vi "drivePID.vi"() -> ()   [LabVIEW 2013]
uses:
  State_Machine_Enum.ctl
  PCQueueDashboard/DBNameEnum.ctl
  RefnameEnum.ctl
  Robot Global Data.vi
  <vilib>/Rock Robotics/WPI/RobotDrive/WPI_RobotDriveGetSetRefNum.vi
panel:
  out "Loop Difference":u32
  in  "RPMRight":dbl(slide)=50.0 min=0.0 max=75.0 step=1.0 scale=0.0..75.0
  in  "RPMLeft":dbl(slide)=50.0 min=0.0 max=75.0 step=1.0 scale=0.0..75.0
  in  "output range RIGHT":cluster{"output high":dbl, "output low":dbl}={"output high"=1.0, "output low"=-1.0} {"output low" min=-1.0 max=1.0 step=0.1 format="%.2f"; "output high" min=-1.0 max=1.0 step=0.1 format="%.2f"}
  in  "output range LEFT":cluster{"output high":dbl, "output low":dbl}={"output high"=1.0, "output low"=-1.0} {"output low" min=-1.0 max=1.0 step=0.1 format="%.2f"; "output high" min=-1.0 max=1.0 step=0.1 format="%.2f"}
  in  "PID RIGHT":T1={"proportional gain (Kc)"=0.015, "integral time (Ti, min)"=0.001, "derivative time (Td, min)"=0.0} {"derivative time (Td, min)" format="%.3f"; "integral time (Ti, min)" format="%.3f"; "proportional gain (Kc)" format="%.3f"}
  in  "PID LEFT":T1={"proportional gain (Kc)"=0.015, "integral time (Ti, min)"=0.001, "derivative time (Td, min)"=0.0} {"derivative time (Td, min)" format="%.3f"; "integral time (Ti, min)" format="%.3f"; "proportional gain (Kc)" format="%.3f"}
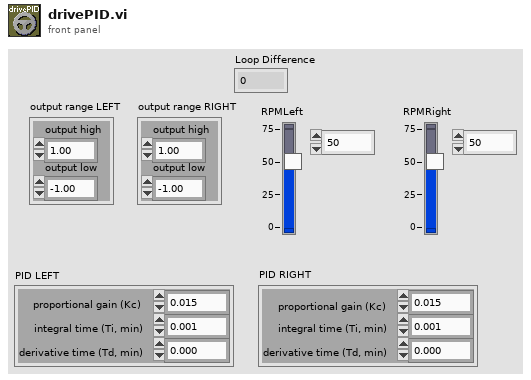
[diagram p1: front panel]
types:
  T1 = cluster{"proportional gain (Kc)":dbl, "integral time (Ti, min)":dbl, "derivative time (Td, min)":dbl}
  T2 = typedef "State_Machine_Enum.ctl" = enum16{"Idle", "Start", "Do", "Stop", "Init"}
  T3 = typedef "DBNameEnum.ctl" = enum16{"AutoInstructions", "DriveLoopTime", "DriveAlignLSLeft", "DriveAlignLSRight", "Use2DriveAlign", "ClimbLS", "LauncherAngleMatches", "FrameworkVersion", "sLauncherAngle", "LauncherTargetAngle", "sLauncherRPM", "LauncherTargetRPM", "sDriveDistance", "LauncherMotorValue", "PullbackTol", "FireTol", "LauncherRPMTol", "LauncherAngleTol", "InitialWait", "WaitBetweenLaunch", "AnglePresets", "RPMPresets", "UseAngleEncoder", "UseLauncherEncoder", "UseLauncherPID", "QSWaitBeforeFire", "QSWaitBeforeRetract", "AngleForwardValue", "AngleBackwardValue", "UseClusterArray", "BackupAuto", "ReverseDriveIndicate", "HalfSpeedFactor"}
  T4 = typedef "RefnameEnum.ctl" = enum16{"FireLauncher", "Climber", "Shield", "TankDrive", "DriveEncoderL", "DriveEncoderR", "LauncherMotorRPM", "LauncherEncoderAnalog", "LauncherEncoderRPM", "ShooterLS", "DriveAlignLSLeft", "DriveAlignLSRight", "ClimbingLS", "LauncherEncoderAngle", "LauncherMotorAngle", "Gamepad1", "Gamepad2", "Compressor", "ClimbWeightSol3", "ClimbWeightSol4"}
  T5 = typedef "WPI_DigitalInputDevRef.ctl" = cluster{"DevStatus":errorcluster, "DIO Channel":T6, "Digital Module":T7}
  T6 = typedef "FPGA_DIOChannel.ctl" = enum8{"DIO 1", "DIO 2", "DIO 3", "DIO 4", "DIO 5", "DIO 6", "DIO 7", "DIO 8", "DIO 9", "DIO 10", "DIO 11", "DIO 12", "DIO 13", "DIO 14", "Invalid"}
  T7 = typedef "FPGA_TypedefDigitalModule.ctl" = enum16{"Digital Module 1", "Digital Module 2"}
  T8 = typedef "WPI_RobotDriveDevRef.ctl" = cluster{"DevStatus":errorcluster, "Motors[]":T9[], "Square Inputs":bool, "Max Output":dbl, "Isochronous":bool}
  T9 = typedef "WPI_MotorControlDeviceRef.ctl" = cluster{"DeviceStatus":errorcluster, "Type":enum16{"PWM", "CAN"}, "PWM":cluster{"Digital Module":T7, "PWM Channel":T10, "DeadBand":T11}, "CAN":cluster{"Device Number":u8, "Control Mode":T12, "Semaphore":T13, "Max Vout":dbl}, "Invert":bool, "TransformRef":T14, "InvTransformRef":T14}
  T10 = typedef "FPGA_DIOPWMChannel.ctl" = enum8{"PWM 1", "PWM 2", "PWM 3", "PWM 4", "PWM 5", "PWM 6", "PWM 7", "PWM 8", "PWM 9", "PWM 10", "Invalid"}
  T11 = typedef "WPI_PWMDeadband.ctl" = cluster{"Name":string, "maxPositivePwm":i32, "minPositivePwm":i32, "centerPwm":i32, "maxNegativePwm":i32, "minNegativePwm":i32, "angularRange":u16}
  T12 = typedef "WPI_CANJaguar_ControlMode.ctl" = enum8{"Percent VBus", "Current", "Speed", "Position", "Voltage"}
  T13 = typedef "Semaphore RefNum" = refnum<k1>
  T14 = typedef "WPI_PWMTransform_ConPane.ctl" = refnum<vi>
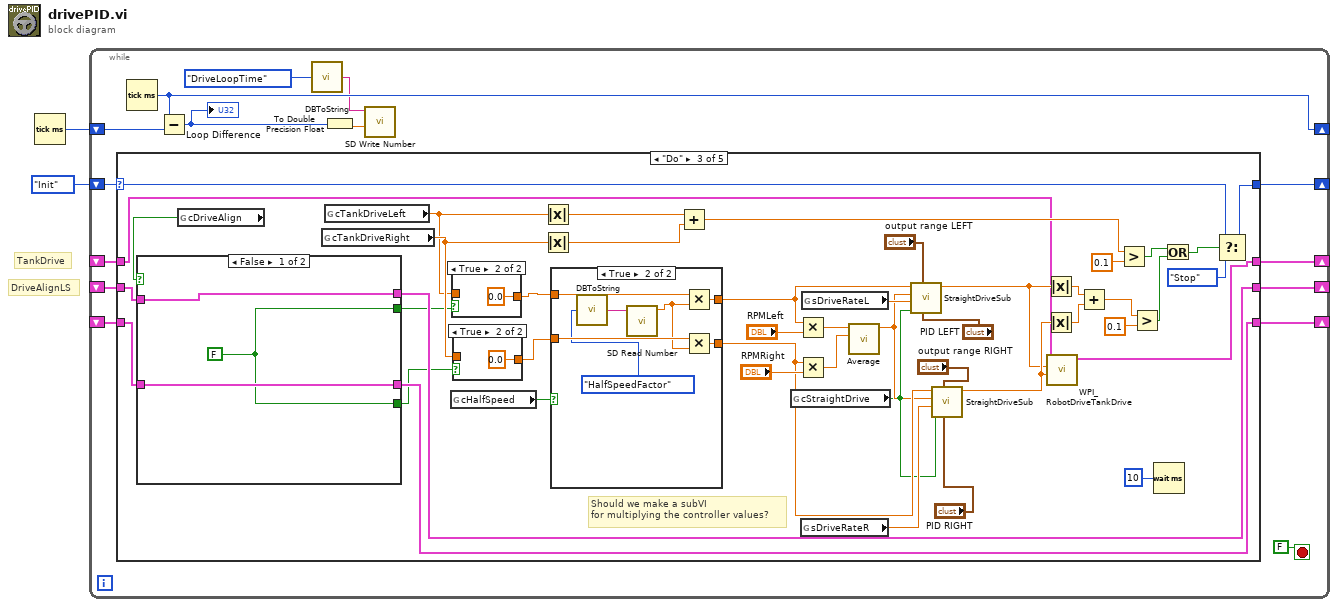
[diagram p0: block diagram]
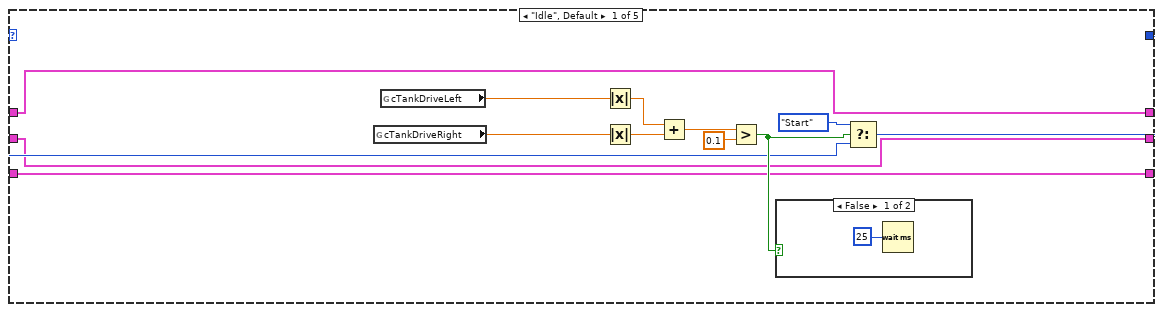
[diagram p2: hidden frame]
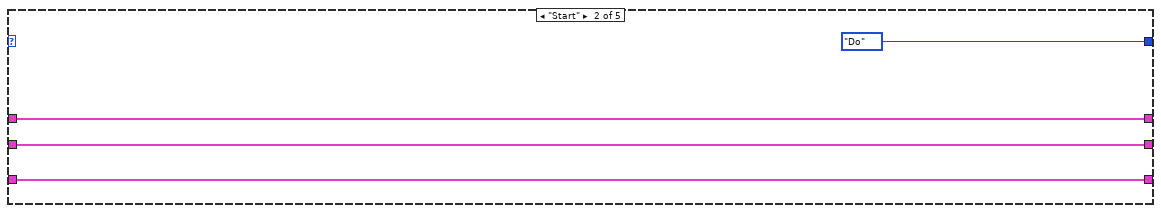
[diagram p4: hidden frame]
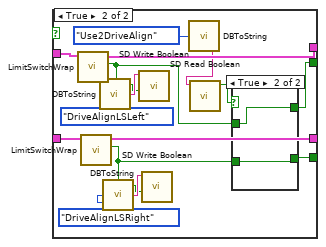
[diagram p7: hidden frame]
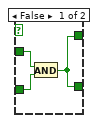
[diagram p8: hidden frame]
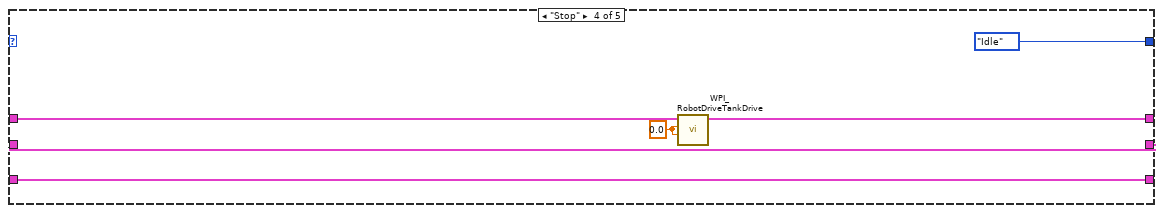
[diagram p10: hidden frame]
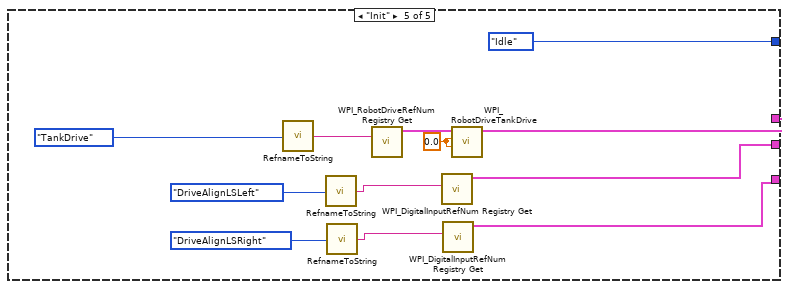
[diagram p11: hidden frame]
diagram:
  # "TankDrive"
  # "DriveAlignLS"
  n1 = Tick Count (ms)() -> (millisecond timer value=w1:u32)
  n2 = while {
    shift-right: [w15] -> _
    shift-left: State_Machine_Enum."Init" ("State") -> [w14]
    shift-right: [w16] -> _
    shift-left: _ -> [w17]
    shift-right: [w10] -> _
    shift-left: w1 -> [w9]
    shift-right: [w8] -> _
    shift-left: _ -> [w7]
    shift-right: [w4] -> _
    shift-left: _ -> [w3]
    stop <- FALSE stop-if-true
    n3 = case shown="\"Do\"" w14 {
      selector: w14 -> [w21 _ w76 _ _]
      tunnel: w17 -> [w20 w35 w46 w122 _]
      tunnel: [w20 w35 w43 w121 w132] -> w16
      tunnel: [w22 State_Machine_Enum."Do" ("State") w77 State_Machine_Enum."Idle" ("State") State_Machine_Enum."Idle" ("State")] -> w15
      tunnel: [w19 w33 w44 w118 w130] -> w8
      tunnel: w7 -> [w19 w33 w48 w118 _]
      tunnel: [w18 w32 w42 w117 w123] -> w4
      tunnel: w3 -> [w18 w32 w45 w117 _]
      frame "Idle", Default {
        n4 = global read "Robot Global Data.vi" "cTankDriveRight"() -> (w25:dbl)
        n5 = global read "Robot Global Data.vi" "cTankDriveLeft"() -> (w26:dbl)
        n6 = Absolute Value(x=w26) -> (abs(x)=w30:dbl)
        n7 = Absolute Value(x=w25) -> (abs(x)=w29:dbl)
        n8 = Add(x=w30, y=w29) -> (x+y=w28:dbl)
        n9 = Greater?(x=w28, y=0.1) -> (0:w23:bool)
        n10 = case shown="False" w23 {
          frame False {
            n11 = Wait (ms)(milliseconds to wait=u32 25) -> ()  [unwired: 1 out]
          }
          frame True {
          }
        }
        n12 = Select(t=State_Machine_Enum."Start" ("State"), s=w23, f=w21) -> (s? t:f=w22:T2)
      }
      frame "Start" {
      }
      frame "Do" {
        # "Should we make a subVI\nfor multiplying the controller values?"
        n13 = global read "Robot Global Data.vi" "cDriveAlign"() -> (w49:bool)
        n14 = case shown="False" w49 {
          tunnel: w48 -> [w87 w102]
          tunnel: [w87 w101] -> w44
          tunnel: w45 -> [w86 w98]
          tunnel: [w86 w97] -> w42
          tunnel: [w85 w89] -> w37
          tunnel: [w85 w88] -> w36
          frame False {
            w85 = FALSE ("Triggered")
          }
          frame True {
            n15 = call "LimitSwitchWrap.vi"("DigitalInputDevRef"=w102) -> ("Triggered"=w91:bool, "DigitalInputDevRef 2"=w101:T5)  [unwired: 9 in]
            n16 = call "LimitSwitchWrap.vi"("DigitalInputDevRef"=w98) -> ("Triggered"=w90:bool, "DigitalInputDevRef 2"=w97:T5)  [unwired: 9 in]
            n17 = call "DBToString.vi"("Enum"=DBNameEnum."DriveAlignLSLeft") -> ("Refname"=w99:string)
            n18 = call "DBToString.vi"("Enum"=DBNameEnum."DriveAlignLSRight") -> ("Refname"=w96:string)
            n19 = call <vilib>:"SD Write Boolean.vi"("Boolean"=w91, "Name"=w99) -> ()  [unwired: 8 in, 2 out]
            n20 = call <vilib>:"SD Write Boolean.vi"("Boolean"=w90, "Name"=w96) -> ()  [unwired: 8 in, 2 out]
            n21 = call "DBToString.vi"("Enum"=DBNameEnum."Use2DriveAlign") -> ("Refname"=w93:string)
            n22 = call <vilib>:"SD Read Boolean.vi"("Name"=w93) -> ("Boolean"=w92:bool)  [unwired: 8 in, 2 out]
            n23 = case shown="True" w92 {
              tunnel: w91 -> [w105 w107]
              tunnel: w90 -> [w104 w106]
              tunnel: [w103 w107] -> w89
              tunnel: [w103 w106] -> w88
              frame False {
                n24 = And(x=w105, y=w104) -> (x .and. y?=w103:bool)
              }
              frame True {
              }
            }
          }
        }
        n25 = global read "Robot Global Data.vi" "cTankDriveRight"() -> (w40:dbl)
        n26 = global read "Robot Global Data.vi" "cTankDriveLeft"() -> (w39:dbl)
        n27 = global read "Robot Global Data.vi" "cHalfSpeed"() -> (w50:bool)
        n28 = case shown="True" w37 {
          tunnel: [w83 0.0 ("cTankDriveLeft")] -> w41
          tunnel: w39 -> [w83 _]
          frame False {
          }
          frame True {
          }
        }
        n29 = case shown="True" w36 {
          tunnel: [w81 0.0 ("cTankDriveLeft")] -> w38
          tunnel: w40 -> [w81 _]
          frame False {
          }
          frame True {
          }
        }
        n30 = Absolute Value(x=w39) -> (abs(x)=w54:dbl)
        n31 = Absolute Value(x=w40) -> (abs(x)=w53:dbl)
        n32 = case shown="True" w50 {
          tunnel: w38 -> [w108 w115]
          tunnel: w41 -> [w109 w116]
          tunnel: [w109 w113] -> w59
          tunnel: [w108 w114] -> w66
          frame False {
          }
          frame True {
            n33 = call "DBToString.vi"("Enum"=DBNameEnum."HalfSpeedFactor") -> ("Refname"=w112:string)
            n34 = call <vilib>:"SD Read Number.vi"("Name"=w112) -> ("Numeric"=w111:dbl)  [unwired: 8 in, 2 out]
            n35 = Multiply(x=w116, y=w111) -> (x*y=w113:dbl)
            n36 = Multiply(x=w115, y=w111) -> (x*y=w114:dbl)
          }
        }
        n37 = Add(x=w54, y=w53) -> (x+y=w55:dbl)
        n38 = global read "Robot Global Data.vi" "cStraightDrive"() -> (w60:bool)
        n39 = Multiply(x=w59, y="RPMLeft") -> (x*y=w80:dbl)
        n40 = Multiply(x=w66, y="RPMRight") -> (x*y=w79:dbl)
        n41 = global read "Robot Global Data.vi" "sDriveRateR"() -> (w67:dbl)
        n42 = global read "Robot Global Data.vi" "sDriveRateL"() -> (w62:dbl)
        n43 = call "Average.vi"("y"=w79, "x"=w80) -> ("x/y"=w61:dbl)  [unwired: 9 in]
        n44 = call "StraightDriveSub.vi"("PID Constants"="PID LEFT", "output range"="output range LEFT", "StraightDriveEngage?"=w60, "sDriveRate"=w62, "Average Controller Value"=w61, "Controller Value"=w59) -> ("Motor Value"=w58:dbl)  [unwired: 5 in]
        n45 = call "StraightDriveSub.vi"("PID Constants"="PID RIGHT", "output range"="output range RIGHT", "StraightDriveEngage?"=w60, "sDriveRate"=w67, "Average Controller Value"=w61, "Controller Value"=w66) -> ("Motor Value"=w65:dbl)  [unwired: 5 in]
        n46 = Absolute Value(x=w58) -> (abs(x)=w70:dbl)
        n47 = Absolute Value(x=w65) -> (abs(x)=w69:dbl)
        n48 = call <vilib>:"WPI_RobotDriveTankDrive.vi"("Right axis value"=w65, "Left axis value"=w58, "RobotDriveDevRef"=w46) -> ("RobotDriveDevRef"=w43:T8)  [unwired: 6 in, 2 out]
        n49 = Add(x=w70, y=w69) -> (x+y=w71:dbl)
        n50 = Greater?(x=w55, y=0.1) -> (0:w51:bool)
        n51 = Greater?(x=w71, y=0.1) -> (0:w52:bool)
        n52 = Wait (ms)(milliseconds to wait=u32 10) -> ()  [unwired: 1 out]
        n53 = Or(x=w51, y=w52) -> (x .or. y?=w68:bool)
        n54 = Select(t=w76, s=w68, f=State_Machine_Enum."Stop") -> (s? t:f=w77:T2)
      }
      frame "Stop" {
        w120 = 0.0 ("Right axis value")
        n55 = call <vilib>:"WPI_RobotDriveTankDrive.vi"("Right axis value"=w120, "Left axis value"=w120, "RobotDriveDevRef"=w122) -> ("RobotDriveDevRef"=w121:T8)  [unwired: 6 in, 2 out]
      }
      frame "Init" {
        w133 = 0.0 ("Left axis value")
        n56 = call "RefnameToString.vi"("Enum"=RefnameEnum."TankDrive") -> ("Refname"=w128:string)
        n57 = call "RefnameToString.vi"("Enum"=RefnameEnum."DriveAlignLSLeft") -> ("Refname"=w126:string)
        n58 = call "RefnameToString.vi"("Enum"=RefnameEnum."DriveAlignLSRight") -> ("Refname"=w125:string)
        n59 = call <vilib>:"WPI_RobotDriveRefNum Registry Get.vi"("refnum name"=w128) -> ("RobotDriveDevRef"=w134:T8)  [unwired: 9 in, 1 out]
        n60 = call <vilib>:"WPI_DigitalInputRefNum Registry Get.vi"("refnum name"=w126) -> ("DigitalInputDevRef"=w130:T5)  [unwired: 9 in, 1 out]
        n61 = call <vilib>:"WPI_DigitalInputRefNum Registry Get.vi"("refnum name"=w125) -> ("DigitalInputDevRef"=w123:T5)  [unwired: 9 in, 1 out]
        n62 = call <vilib>:"WPI_RobotDriveTankDrive.vi"("Right axis value"=w133, "Left axis value"=w133, "RobotDriveDevRef"=w134) -> ("RobotDriveDevRef"=w132:T8)  [unwired: 6 in, 2 out]
      }
    }
    n63 = Tick Count (ms)() -> (millisecond timer value=w10:u32)
    n64 = Subtract(x=w10, y=w9) -> (x-y=w12:u32)
    "Loop Difference" <- w12
    n65 = call "DBToString.vi"("Enum"=DBNameEnum."DriveLoopTime") -> ("Refname"=w5:string)
    n66 = To Double Precision Float(number=w12) -> (double precision float=w11:dbl)
    n67 = call <vilib>:"SD Write Number.vi"("Numeric"=w11, "Name"=w5) -> ()  [unwired: 8 in, 2 out]
  }
